vi "Read Column Factory Type.vi"(8 "error in (no error)":errorcluster, 11 "Table Configuration in":refnum<class "Table Configuration.lvclass">) -> (0 "error out":errorcluster, 2 "Basic Columns.lvlib:Basic Column Factory.lvclass":refnum<class "Basic Column Factory.lvclass">, 3 "Table Configuration out":refnum<class "Table Configuration.lvclass">)   [LabVIEW 2020, in "Table.lvlib" / "Table Configuration.lvclass"]
uses:
  Table Configuration.lvclass
  Column Libraries/Basic Columns/Column Configuration/Basic Column Factory Class/Basic Column Factory.lvclass
  Table Configuration.lvclass/Table Configuration.ctl
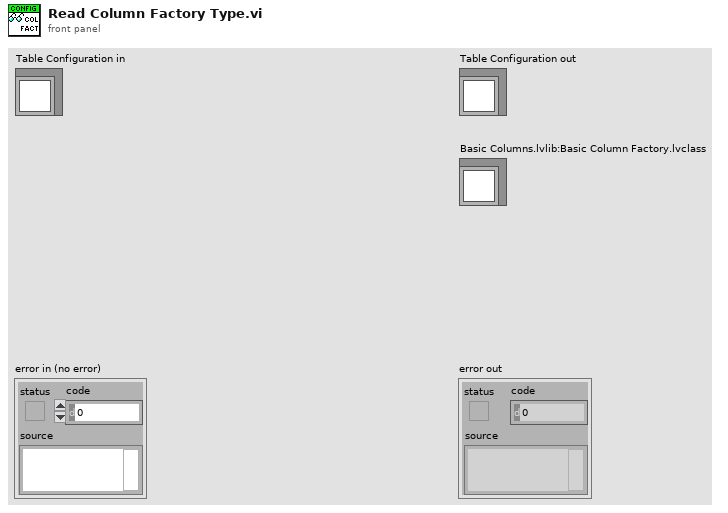
[diagram p1: front panel]
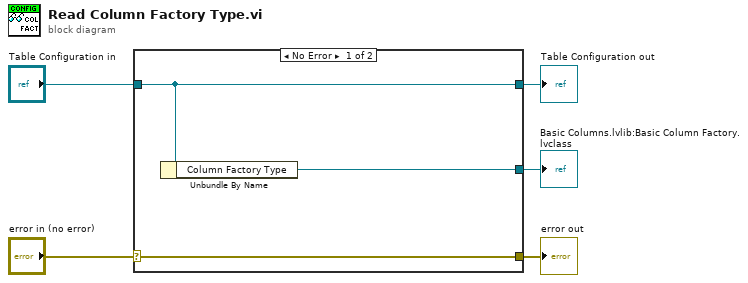
[diagram p0: block diagram]
diagram:
  n1 = case shown="No Error" "error in (no error)" {
    selector: "error in (no error)" -> [w8 w9]
    tunnel: [w8 w9] -> w4
    tunnel: [w7 w10] -> w2
    tunnel: "Table Configuration in" -> [w7 w10]
    tunnel: [w6 _] -> w1
    frame No Error {
      n2 = Unbundle By Name(w7) -> ("Column Factory Type"=w6:refnum<class "Basic Column Factory.lvclass">)
    }
    frame Error {
    }
  }
  "error out" <- w4
  "Table Configuration out" <- w2
  "Basic Columns.lvlib:Basic Column Factory.lvclass" <- w1
